vi "Stop Core.vi"(10 "final error code":i32, 11 "Universal Power Meter in":refnum<class "Universal Power Meter.lvclass">) -> (3 "Universal Power Meter out":refnum<class "Universal Power Meter.lvclass">)   [LabVIEW 2014, in "Universal Power Meter.lvlib" / "Universal Power Meter.lvclass"]
doc: "(<B>Filename</B>: Actor Framework.lvlib:Actor.lvclass:Stop Core.vi)\n\nDefines what the actor does before it stops. Use the <B>final error code</B> input to determine whether the actor shut down in response to an error.\n\nBy default, this method does nothing. A descendant class may override it to define behavior, such as shutting down any processes the actor initiated in its override of the Actor Core method."
uses:
  Universal Power Meter.lvclass
  <vilib>/ActorFramework/Actor/Actor.lvclass
panel:
  out "error out":errorcluster
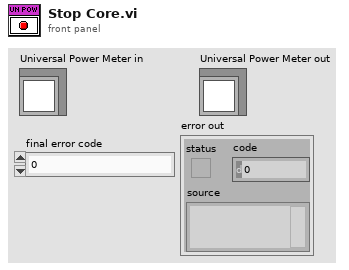
[diagram p1: front panel]
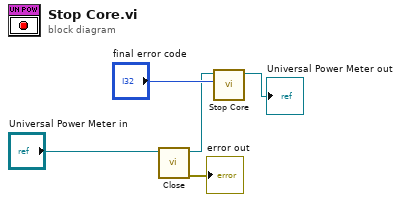
[diagram p0: block diagram]
diagram:
  n1 = call-dynamic "Close.vi"("Universal Power Meter in"="Universal Power Meter in") -> ("error out"=→"error out":errorcluster, "Universal Power Meter out"=w2:refnum<class "Universal Power Meter.lvclass">)  [unwired: 8 in, 1 out]
  n2 = call-parent "Stop Core.vi"("final error code"="final error code", "Actor in"=w2) -> ("Actor out"=→"Universal Power Meter out":refnum<class "Universal Power Meter.lvclass">)  [unwired: 9 in]
